vi "冒道.vi"() -> ()   [LabVIEW 2017]
panel:
  out "Out 5":u8 format="%.0x"
  out "Out 4":u8 format="%.0x"
  out "Out 3":u8 format="%.0x"
  out "Out 2":u8 format="%.0x"
  out "Out":u8 format="%.0x"
  in  "address":string="192.168.10.10"
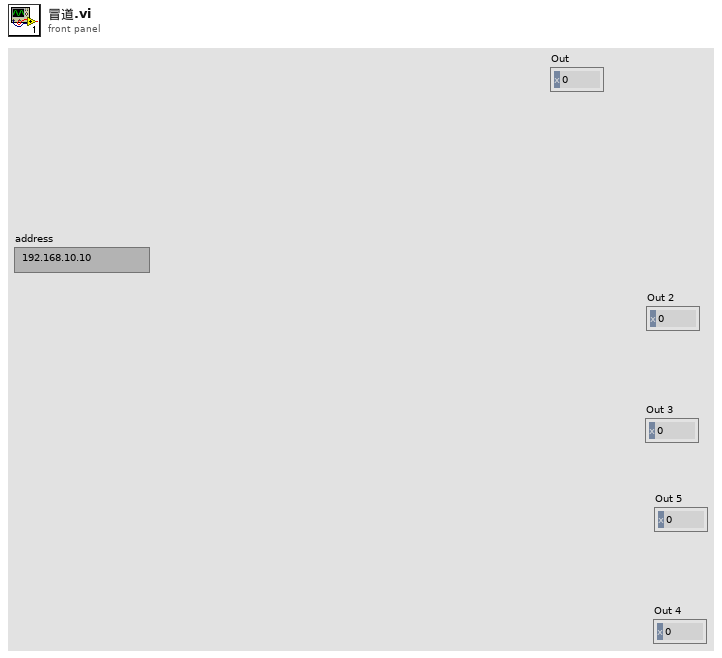
[diagram p1: front panel]
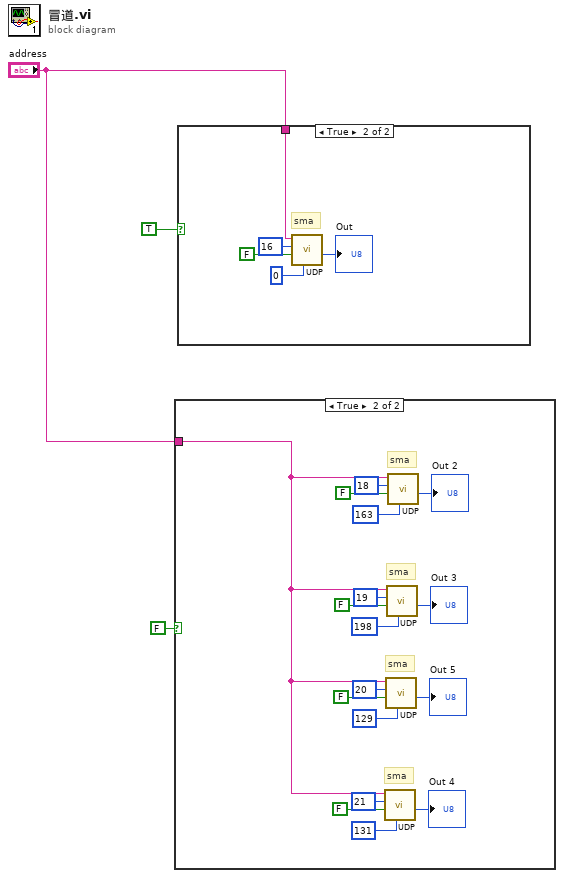
[diagram p0: block diagram]
diagram:
  n1 = case shown="True" FALSE {
    tunnel: "address" -> [_ w4]
    frame False {
    }
    frame True {
      # "sma"
      # "sma"
      # "sma"
      # "sma"
      n2 = call "UDP.vi"("In"=u8 131, "Read (TRUE)"=FALSE, "Address"=u32 21, "IP address"=w4) -> ("Out"=→"Out 4":u8)  [unwired: 5 in, 1 out]
      n3 = call "UDP.vi"("In"=u8 129, "Read (TRUE)"=FALSE, "Address"=u32 20, "IP address"=w4) -> ("Out"=→"Out 5":u8)  [unwired: 5 in, 1 out]
      n4 = call "UDP.vi"("In"=u8 198, "Read (TRUE)"=FALSE, "Address"=u32 19, "IP address"=w4) -> ("Out"=→"Out 3":u8)  [unwired: 5 in, 1 out]
      n5 = call "UDP.vi"("In"=u8 163, "Read (TRUE)"=FALSE, "Address"=u32 18, "IP address"=w4) -> ("Out"=→"Out 2":u8)  [unwired: 5 in, 1 out]
    }
  }
  n6 = case shown="True" TRUE {
    tunnel: "address" -> [_ w21]
    frame False {
    }
    frame True {
      # "sma"
      n7 = call "UDP.vi"("In"=u8 0, "Read (TRUE)"=FALSE, "Address"=u32 16, "IP address"=w21) -> ("Out"=→"Out":u8)  [unwired: 5 in, 1 out]
    }
  }
